vi "Deadzone.vi"(8 "error in (no error)":errorcluster, 9 "Deadzone":dbl, 10 "Input":dbl) -> (0 "error out":errorcluster, 1 "Just entered deadzone?":bool, 2 "In deadzone?":bool)   [LabVIEW 2014]
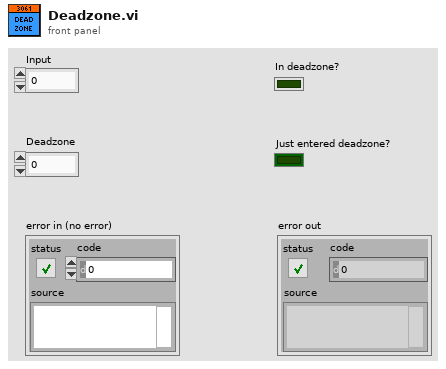
[diagram p1: front panel]
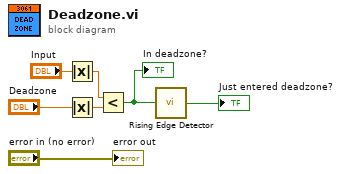
[diagram p0: block diagram]
diagram:
  n1 = Absolute Value(x="Input") -> (abs(x)=w6:dbl)
  n2 = Absolute Value(x="Deadzone") -> (abs(x)=w4:dbl)
  n3 = Less?(x=w6, y=w4) -> (x < y?=w2:bool)
  "In deadzone?" <- w2
  n4 = call "Rising Edge Detector.vi"("Input"=w2) -> ("Rising edge?"=→"Just entered deadzone?":bool)
  "error out" <- "error in (no error)"
